vi "Write Event to Log.vi"(8 "error in (no error)":errorcluster, 9 "Log Event Details":string="Input Log Details", 10 "Enum":enum16{"Event", "Error"}(ring), 11 "Actor_log in":refnum<class "Actor_log.lvclass">) -> (0 "error out":errorcluster, 3 "Actor_log out":refnum<class "Actor_log.lvclass">)   [LabVIEW 2020, in "Actor_log.lvlib" / "Actor_log.lvclass"]
uses:
  Actor_log.lvclass
  Actor_log.lvclass/Actor_log.ctl
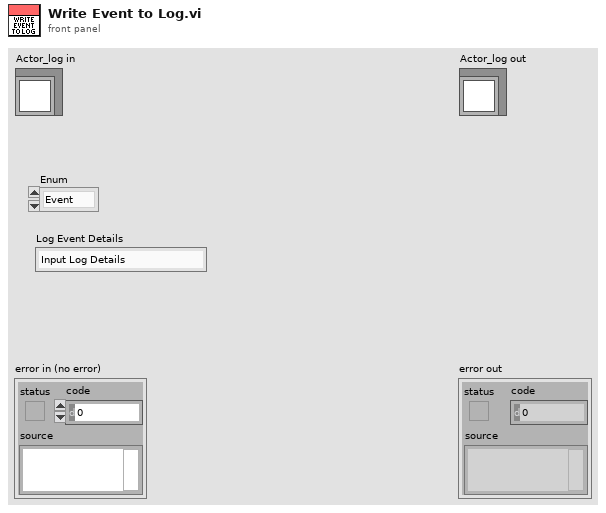
[diagram p1: front panel]
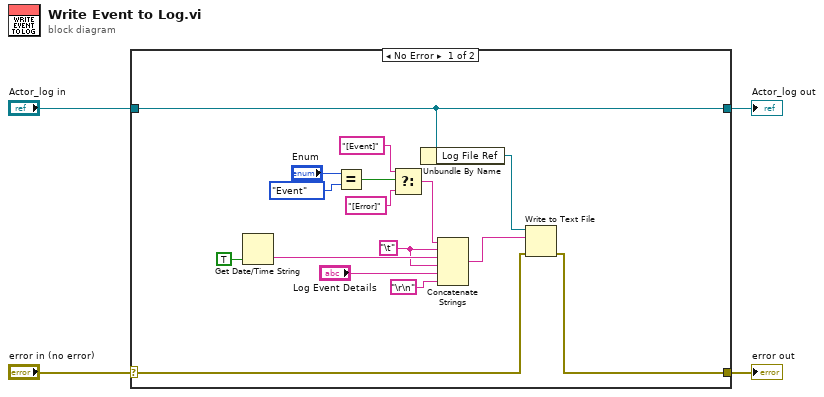
[diagram p0: block diagram]
diagram:
  n1 = case shown="No Error" "error in (no error)" {
    selector: "error in (no error)" -> [w6 w22]
    tunnel: [w5 w22] -> w3
    tunnel: [w10 w21] -> w1
    tunnel: "Actor_log in" -> [w10 w21]
    frame No Error {
      w18 = "\t"
      n2 = Get Date/Time String(want seconds? (F)=TRUE) -> (time string=w19:string)  [unwired: 2 in, 1 out]
      n3 = Equal?(x="Enum", y=enum16{"Event", "Error"}."Event") -> (x = y?=w14:bool)
      n4 = Select(t="[Event]" ("string"), s=w14, f="[Error]" ("string")) -> (s? t:f=w11:string)
      n5 = Unbundle By Name(w10) -> ("Log File Ref"=w8:refnum<file>)
      n6 = Concatenate Strings(w11, w18, w19, w18, "Log Event Details", "\r\n") -> (w7:string)
      n7 = Write to Text File(file (use dialog)=w8, text=w7, error in=w6) -> (error out=w5:errorcluster)  [unwired: 1 in, 2 out]
    }
    frame Error {
    }
  }
  "error out" <- w3
  "Actor_log out" <- w1
